vi "AnAlyZEPoINting_SuBVi.vi"(9 "Array in":dbl[][](array[numeric]), 10 "file name":string, 11 "WaveformGraph in":refnum<vi>) -> (1 "Array out":dbl[][](array[numeric]), 2 "standard deviation 2":dbl format="%0.2f", 3 "new picture":picture, 4 "Plot Images:Front 2":picture, 5 "standard deviation total":dbl format="%0.2f", 6 "standard deviation":dbl format="%0.2f", 7 "Waveform Graph":dbl[][](graph))   [LabVIEW 2011]
uses:
  <vilib>/Analysis/NI_AALBase.lvlib
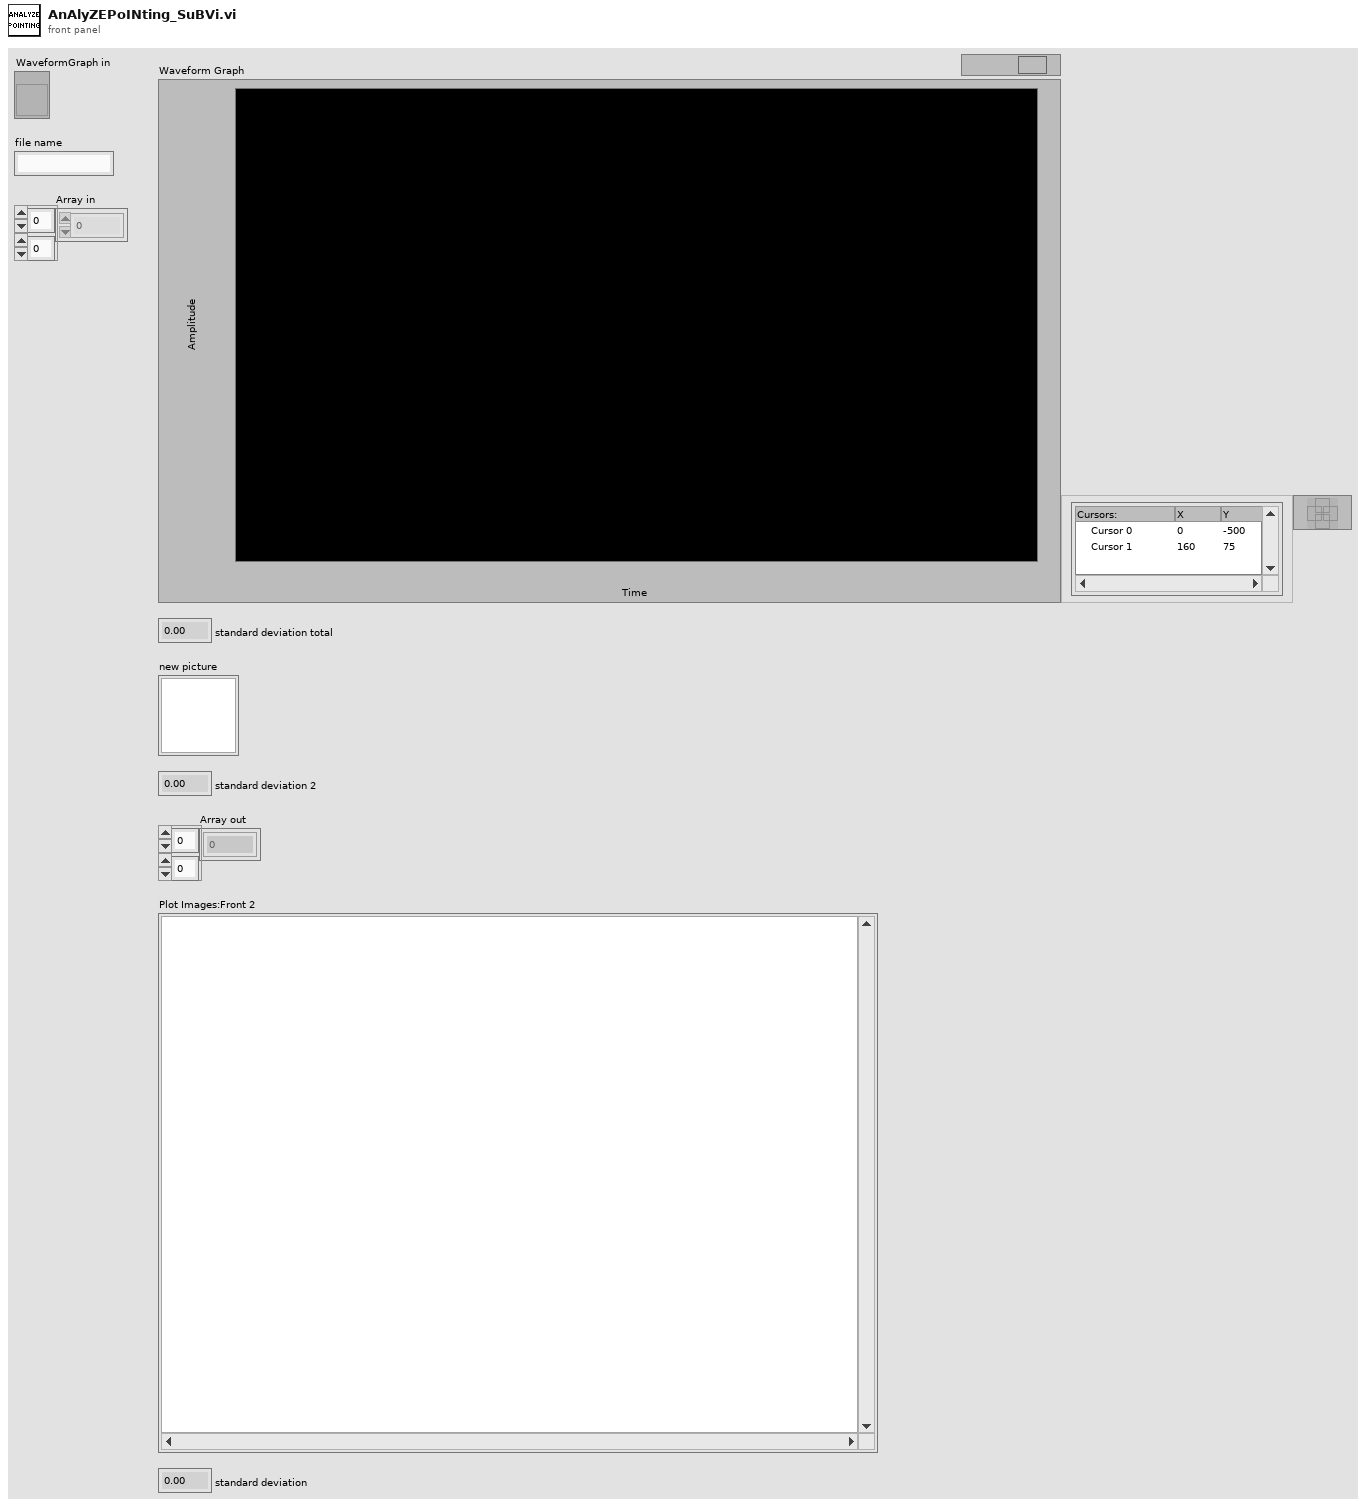
[diagram p1: front panel]
types:
  T1 = cluster{"Width":u16, "Style":enum32{"Solid", "Dash", "Dot", "DashDot", "DashDotDot"}}
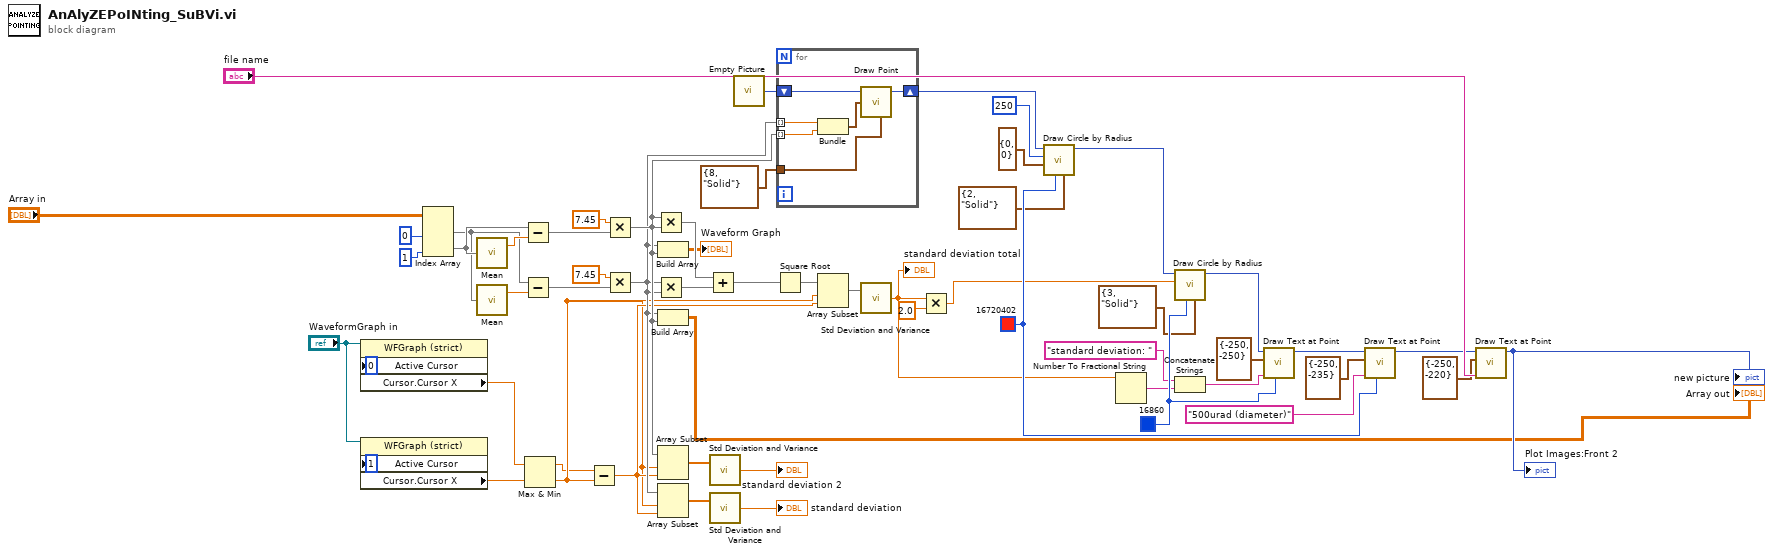
[diagram p0: block diagram]
diagram:
  w46 = u32 16860 ("color(black)")
  w49 = u32 16720402 ("color(black)")
  n1 = property on="Property Node" class="WFGraph (strict)"(reference="WaveformGraph in", "Active Cursor"=u32 0) -> ("Cursor.Cursor X"=w15:dbl)  [unwired: 1 in, 2 out]
  n2 = property on="Property Node" class="WFGraph (strict)"(reference="WaveformGraph in", "Active Cursor"=u32 1) -> ("Cursor.Cursor X"=w16:dbl)  [unwired: 1 in, 2 out]
  n3 = Index Array(array="Array in", index (col) #1=0 ("disabled index (col)"), index (col) #2=1 ("index (col)")) -> (element #1=w4:dbl[], element #2=w7:dbl[])  [unwired: 2 in]
  n4 = call <vilib>:"Mean.vi"("X"=w7) -> ("mean"=w6:dbl)  [unwired: 1 out]
  n5 = call <vilib>:"Mean.vi"("X"=w4) -> ("mean"=w5:dbl)  [unwired: 1 out]
  n6 = Subtract(x=w7, y=w6) -> (x-y=w11:dbl[])
  n7 = Subtract(x=w4, y=w5) -> (x-y=w9:dbl[])
  n8 = Max & Min(x=w15, y=w16) -> (max(x,y)=w17:dbl, min(x,y)=w27:dbl)
  n9 = Subtract(x=w17, y=w27) -> (x-y=w28:dbl)
  n10 = Multiply(x=7.45, y=w11) -> (x*y=w52:dbl[])
  n11 = Multiply(x=7.45, y=w9) -> (x*y=w51:dbl[])
  n12 = Multiply(x=w52, y=w52) -> (x*y=w23:dbl[])
  n13 = Multiply(x=w51, y=w51) -> (x*y=w24:dbl[])
  n14 = Build Array(w51, w52) -> (→"Waveform Graph":dbl[][])
  n15 = Build Array(w51, w52) -> (→"Array out":dbl[][])
  n16 = Array Subset(array=w52, index=w27, length=w28) -> (w20:dbl[])
  n17 = Array Subset(array=w51, index=w27, length=w28) -> (w18:dbl[])
  n18 = Add(x=w23, y=w24) -> (x+y=w25:dbl[])
  n19 = call <vilib>:"Std Deviation and Variance.vi"("X"=w20) -> ("standard deviation"=→"standard deviation 2":dbl)  [unwired: 1 in, 2 out]
  n20 = call <vilib>:"Std Deviation and Variance.vi"("X"=w18) -> ("standard deviation"=→"standard deviation":dbl)  [unwired: 1 in, 2 out]
  n21 = call "Empty Picture"() -> ("empty picture"=w30:picture)
  n22 = Square Root(x=w25) -> (sqrt(x)=w26:dbl[])
  n23 = for {
    tunnel: w51 -> [w63] mode=indexing
    tunnel: w52 -> [w62] mode=indexing
    shift-right: [w59] -> w31
    shift-left: w30 -> [w60]
    tunnel: T1 {"Width"=8, "Style"=enum."Solid"} ("pen") -> [w58]
    n24 = Bundle(w63, w62) -> (w61:cluster{dbl, dbl})  [unwired: 1 in]
    n25 = call <vilib>:"Draw Point.vi"("picture"=w60, "point(x,y)"=w61, "pen"=w58) -> ("new picture"=w59:picture)  [unwired: 6 in]
  }
  n26 = Array Subset(array=w26, index=w27, length=w28) -> (w29:dbl[])
  n27 = call <vilib>:"Std Deviation and Variance.vi"("X"=w29) -> ("standard deviation"=w42:dbl)  [unwired: 1 in, 2 out]
  "standard deviation total" <- w42
  n28 = Multiply(x=w42, y=2.0) -> (x*y=w39:dbl)
  n29 = call <vilib>:"Draw Circle by Radius.vi"("pen"=T1 {"Width"=2, "Style"=enum."Solid"}, "color(black)"=w49, "pixel center"=cluster{"horizontal":i16, "vertical":i16} {"horizontal"=0, "vertical"=0}, "radius"=i16 250, "picture"=w31) -> ("new picture"=w36:picture)  [unwired: 6 in]
  n30 = Number To Fractional String(number=w42) -> (F-format string=w43:string)  [unwired: 3 in]
  n31 = call <vilib>:"Draw Circle by Radius.vi"("pen"=T1 {"Width"=3, "Style"=enum."Solid"}, "color(black)"=w46, "radius"=w39, "picture"=w36) -> ("new picture"=w40:picture)  [unwired: 7 in]
  n32 = Concatenate Strings("standard deviation: " ("text"), w43) -> (w44:string)
  n33 = call <vilib>:"Draw Text at Point.vi"("text color(black)"=w46, "text"=w44, "origin"=cluster{"x":i16, "y":i16} {"x"=-250, "y"=-250}, "picture"=w40) -> ("new picture"=w47:picture)  [unwired: 6 in, 1 out]
  n34 = call <vilib>:"Draw Text at Point.vi"("text color(black)"=w49, "text"="500urad (diameter)", "origin"=cluster{"x":i16, "y":i16} {"x"=-250, "y"=-235}, "picture"=w47) -> ("new picture"=w54:picture)  [unwired: 6 in, 1 out]
  n35 = call <vilib>:"Draw Text at Point.vi"("text"="file name", "origin"=cluster{"x":i16, "y":i16} {"x"=-250, "y"=-220}, "picture"=w54) -> ("new picture"=→"Plot Images:Front 2" →"new picture":picture)  [unwired: 7 in, 1 out]
